vi "Read or Write Dashboard.vi"   [LabVIEW 2016]
uses:
  Global Variables/Sensor Data.vi
  <vilib>/Rock Robotics/Network Tables/NT Write Number.vi
  Global Variables/Robot Status.vi
  <vilib>/Rock Robotics/Network Tables/NT Write Boolean.vi
  Drive and Climb SS/Drive and Climb Logging Values.vi
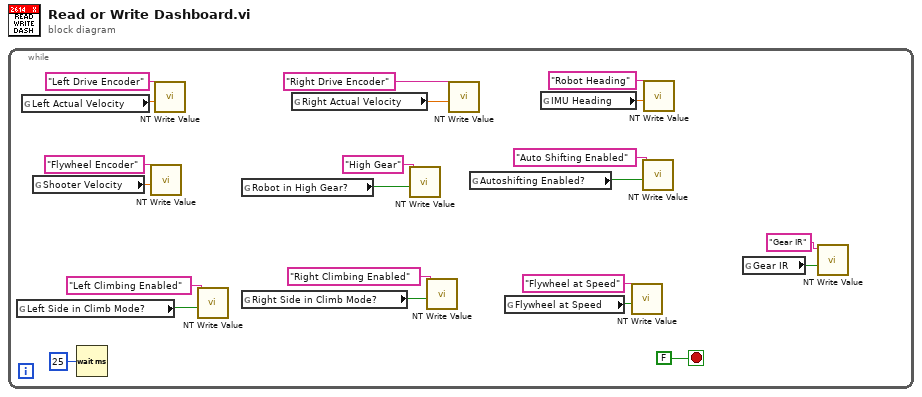
[diagram p0: block diagram]
diagram:
  n1 = while {
    stop <- FALSE stop-if-true
    n2 = global read "Robot Status.vi" "Left Side in Climb Mode?"() -> (w12:bool)
    n3 = global read "Drive and Climb Logging Values.vi" "Left Actual Velocity"() -> (w2:dbl)
    n4 = global read "Sensor Data.vi" "Shooter Velocity"() -> (w16:dbl)
    n5 = Wait (ms)(milliseconds to wait=u32 25) -> ()  [unwired: 1 out]
    n6 = call-poly <vilib>:"NT Write Value.vi"("Numeric"=w16, "Name"="Flywheel Encoder") -> ()  [unwired: 9 in, 1 out]
    n7 = call-poly <vilib>:"NT Write Value.vi"("Numeric"=w2, "Name"="Left Drive Encoder") -> ()  [unwired: 9 in, 1 out]
    n8 = call-poly <vilib>:"NT Write Value.vi"("Boolean"=w12, "Name"="Left Climbing Enabled") -> ()  [unwired: 9 in, 1 out]
    n9 = global read "Robot Status.vi" "Robot in High Gear?"() -> (w8:bool)
    n10 = global read "Robot Status.vi" "Right Side in Climb Mode?"() -> (w9:bool)
    n11 = global read "Drive and Climb Logging Values.vi" "Right Actual Velocity"() -> (w1:dbl)
    n12 = call-poly <vilib>:"NT Write Value.vi"("Boolean"=w8, "Name"="High Gear") -> ()  [unwired: 9 in, 1 out]
    n13 = call-poly <vilib>:"NT Write Value.vi"("Boolean"=w9, "Name"="Right Climbing Enabled") -> ()  [unwired: 9 in, 1 out]
    n14 = call-poly <vilib>:"NT Write Value.vi"("Numeric"=w1, "Name"="Right Drive Encoder") -> ()  [unwired: 9 in, 1 out]
    n15 = global read "Robot Status.vi" "Autoshifting Enabled?"() -> (w5:bool)
    n16 = global read "Robot Status.vi" "Flywheel at Speed"() -> (w14:bool)
    n17 = global read "Sensor Data.vi" "IMU Heading"() -> (w18:dbl)
    n18 = call-poly <vilib>:"NT Write Value.vi"("Boolean"=w14, "Name"="Flywheel at Speed") -> ()  [unwired: 9 in, 1 out]
    n19 = call-poly <vilib>:"NT Write Value.vi"("Boolean"=w5, "Name"="Auto Shifting Enabled") -> ()  [unwired: 9 in, 1 out]
    n20 = call-poly <vilib>:"NT Write Value.vi"("Numeric"=w18, "Name"="Robot Heading") -> ()  [unwired: 9 in, 1 out]
    n21 = global read "Sensor Data.vi" "Gear IR"() -> (w4:bool)
    n22 = call-poly <vilib>:"NT Write Value.vi"("Boolean"=w4, "Name"="Gear IR") -> ()  [unwired: 9 in, 1 out]
  }
